vi "Common Response.vi"(8 "RSP":string, 10 "Data":string) -> (0 "RSPo":string, 1 "unlisted":bool, 2 "Datao":string, 3 "error":string)   [LabVIEW 2019, in "FINS TCP.lvlib"]
uses:
  FINS TCP.lvlib
panel:
  out "RSP length":i32
  out "data length":i32
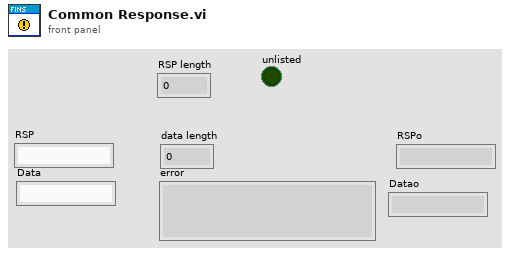
[diagram p1: front panel]
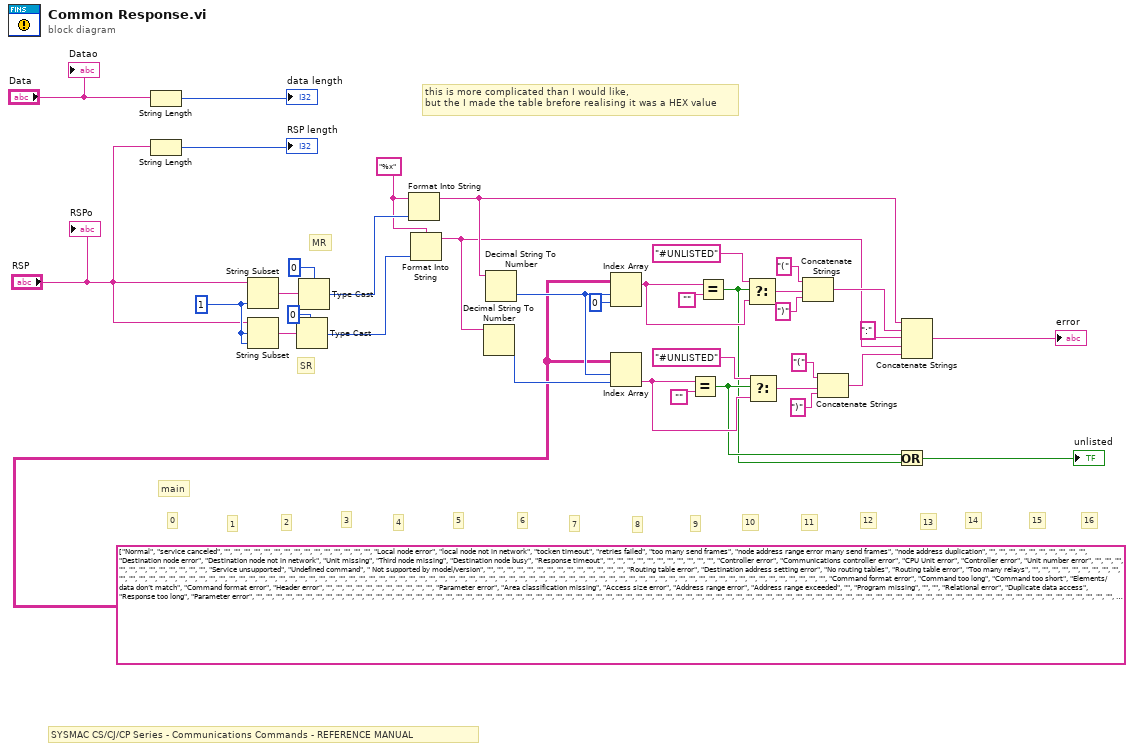
[diagram p0: block diagram]
diagram:
  w16 = string[][] [["Normal", "service canceled", "", "", "", "", "", "", "", "", "", "", "", "", "", "", ""], ["Local node error", "local node not in network", "tocken timeout", "retries failed", "too many send frames", "node address range error many send frames", "node address duplication", "", "", "", "", "", "", "", "", "", ""], ["Destination node error", "Destination node not in network", "Unit missing", "Third node missing", "Destination node busy", "Response timeout", "", "", "", "", "", "", "", "", "", "", ""], ["Controller error", "Communications controller error", "CPU Unit error", "Controller error", "Unit number error", "", "", "", "", "", "", "", "", "", "", "", ""], ["Service unsupported", "Undefined command", " Not supported by model/version", "", "", "", "", "", "", "", "", "", "", "", "", "", ""], ["Routing table error", "Destination address setting error", "No routing tables", "Routing table error", "Too many relays", "", "", "", "", "", "", "", "", "", "", "", ""], ["", "", "", "", "", "", "", "", "", "", "", "", "", "", "", "", ""], ["", "", "", "", "", "", "", "", "", "", "", "", "", "", "", "", ""], ["", "", "", "", "", "", "", "", "", "", "", "", "", "", "", "", ""], ["", "", "", "", "", "", "", "", "", "", "", "", "", "", "", "", ""], ["Command format error", "Command too long", "Command too short", "Elements/ data don’t match", "Command format error", "Header error", "", "", "", "", "", "", "", "", "", "", ""], ["Parameter error", "Area classification missing", "Access size error", "Address range error", "Address range exceeded", "", "Program missing", "", "", "Relational error", "Duplicate data access", "Response too long", "Parameter error", "", "", "", ""], ["", "", "", "", "", "", "", "", "", "", "", "", "", "", "", "", ""], ["", "", "", "", "", "", "", "", "", "", "", "", "", "", "", "", ""], ["", "", "", "", "", "", "", "", "", "", "", "", "", "", "", "", ""], ["", "", "", "", "", "", "", "", "", "", "", "", "", "", "", "", ""], ["", "", "", "", "", "", "", "", "", "", "", "", "", "", "", "", ""], ["", "", "", "", "", "", "", "", "", "", "", "", "", "", "", "", ""], ["", "", "", "", "", "", "", "", "", "", "", "", "", "", "", "", ""], ["", "", "", "", "", "", "", "", "", "", "", "", "", "", "", "", ""], ["Read not possible", "", "Protected", "Table missing", "Data missing", "Program missing", "File missing", "Data mismatch", "", "", "", "", "", "", "", "", ""], ["Write not possible", "Read-only", "Protected", "Cannot register", "", "Program missing", "File missing", "File name already exists", "Cannot change", "", "", "", "", "", "", "", ""], ["Not executable in current mode", "Not possible during execution", "Not possible while running", "Wrong PLC mode", "Wrong PLC mode", "Wrong PLC mode", "Wrong PLC mode", "Specified node not polling node", "Step cannot be executed", "", "", "", "", "", "", "", ""], ["No such device", "File device missing", "Memory missing", "Clock missing", "", "", "", "", "", "", "", "", "", "", "", "", ""], ["Cannot start/stop", "Table missing", "", "", "", "", "", "", "", "", "", "", "", "", "", "", ""], ["Unit error", "", "Memory error", "I/O setting error", "Too many I/O points", "CPU bus error", "I/O duplication", "I/O bus error", "", "SYSMAC BUS/2 error", "CPU Bus Unit error", "", "", "SYSMAC BUS No. duplication", "", "Memory error", "SYSMAC BUS terminator missing"], ["Command error", "No protection", "Incorrect password ", "", "Protected", "Service already executing", " Service stopped", "No execution right", "Settings not complete", "Necessary items not set", "Number already defined", "Error will not clear", "", "", "", "", ""], ["", "", "", "", "", "", "", "", "", "", "", "", "", "", "", "", ""], ["", "", "", "", "", "", "", "", "", "", "", "", "", "", "", "", ""], ["", "", "", "", "", "", "", "", "", "", "", "", "", "", "", "", ""], ["Access right error", "No access right", "", "", "", "", "", "", "", "", "", "", "", "", "", "", ""], ["", "", "", "", "", "", "", "", "", "", "", "", "", "", "", "", ""], ["", "", "", "", "", "", "", "", "", "", "", "", "", "", "", "", ""], ["", "", "", "", "", "", "", "", "", "", "", "", "", "", "", "", ""], ["", "", "", "", "", "", "", "", "", "", "", "", "", "", "", "", ""], ["", "", "", "", "", "", "", "", "", "", "", "", "", "", "", "", ""], ["", "", "", "", "", "", "", "", "", "", "", "", "", "", "", "", ""], ["", "", "", "", "", "", "", "", "", "", "", "", "", "", "", "", ""], ["", "", "", "", "", "", "", "", "", "", "", "", "", "", "", "", ""], ["", "", "", "", "", "", "", "", "", "", "", "", "", "", "", "", ""], ["Abort", "Service aborted", "", "", "", "", "", "", "", "", "", "", "", "", "", "", ""]] ("Array 2")
  w17 = "%x" ("format string")
  w35 = 1 ("length (rest)")
  # "this is more complicated than I would like, \nbut the I made the table brefore realising it was a HEX value"
  # "SYSMAC CS/CJ/CP Series - Communications Commands - REFERENCE MANUAL"
  # "16"
  # "15"
  # "14"
  # "13"
  # "12"
  # "11"
  # "main"
  # "10"
  # "9"
  # "8"
  # "7"
  # "6"
  # "5"
  # "4"
  # "3"
  # "2"
  # "1"
  # "0"
  # "SR"
  # "MR"
  n1 = String Length(string="Data") -> (length=→"data length":i32)
  n2 = String Length(string="RSP") -> (length=→"RSP length":i32)
  n3 = String Subset(string="RSP", length (rest)=w35) -> (substring=w34:string)  [unwired: 1 in]
  n4 = String Subset(string="RSP", offset (0)=w35, length (rest)=w35) -> (substring=w32:string)
  n5 = Type Cast(type=u8 0 ("length (rest)"), x=w32) -> (*(type *) &x=w20:u8)
  n6 = Type Cast(type=u8 0 ("length (rest)"), x=w34) -> (*(type *) &x=w22:u8)
  n7 = Format Into String(format string=w17, w22) -> (resulting string=w15:string)  [unwired: 2 in, 1 out]
  n8 = Format Into String(format string=w17, w20) -> (resulting string=w6:string)  [unwired: 2 in, 1 out]
  n9 = Decimal String To Number(string=w6) -> (number=w18:i32)  [unwired: 2 in, 1 out]
  n10 = Decimal String To Number(string=w15) -> (number=w19:i32)  [unwired: 2 in, 1 out]
  n11 = Index Array(array=w16, index (row)=w19, index (col)=0 ("disabled index (col)")) -> (element=w24:string)
  n12 = Index Array(array=w16, index (row)=w19, index (col)=w18) -> (element=w27:string)
  n13 = Equal?(x=w27, y="") -> (x = y?=w4:bool)
  n14 = Equal?(x=w24, y="") -> (x = y?=w3:bool)
  n15 = Select(t="#UNLISTED" ("name"), s=w3, f=w24) -> (s? t:f=w14:string)
  n16 = Select(t="#UNLISTED" ("name"), s=w4, f=w27) -> (s? t:f=w9:string)
  n17 = Concatenate Strings("(" ("string"), w14, ")" ("string")) -> (w7:string)
  n18 = Concatenate Strings("(" ("string"), w9, ")" ("string")) -> (w8:string)
  n19 = Or(x=w4, y=w3) -> (x .or. y?=→"unlisted":bool)
  n20 = Concatenate Strings(w15, w7, ":" ("string"), w6, w8) -> (→"error":string)
  "Datao" <- "Data"
  "RSPo" <- "RSP"
